vi "Polynomial_Fit.vi"(6 "tolerance":dbl=0.0001, 7 "polynomial order":i32=2, 8 "algorithm":T1 items=["SVD", "Givens", "Givens2", "Householder", "LU Decomposition", "Cholesky", "SVD for Rank Deficient H"], 9 "method":T2 items=["Least Square", "Least Absolute Residual", "Bisquare"], 10 "time":dbl[](array[numeric]), 11 "Y":dbl[](array[numeric])) -> (1 "Polynomial Coefficients":dbl[](array[numeric]), 2 "Equation Y(time)":string, 3 "Plot":cluster{"time":dbl[], "P(A)":dbl[]}[](graph))   [LabVIEW 2022 SP3]
uses:
  <vilib>/Analysis/6fits.llb/Curve Fitting Criteria.ctl
  <vilib>/Analysis/6fits.llb/General Linear Fit Algorithm.ctl
  <vilib>/Analysis/polynomials.llb/Polynomial Plot (Samples).vi
  <vilib>/Analysis/NI_AALPro.lvlib
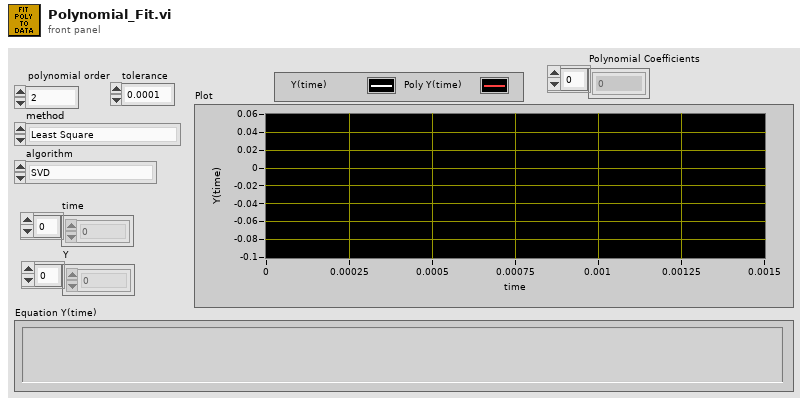
[diagram p1: front panel]
types:
  T1 = typedef "NI_AALPro.lvlib/General Linear Fit Algorithm.ctl" = u16
  T2 = typedef "NI_AALPro.lvlib/Curve Fitting Criteria.ctl" = u16
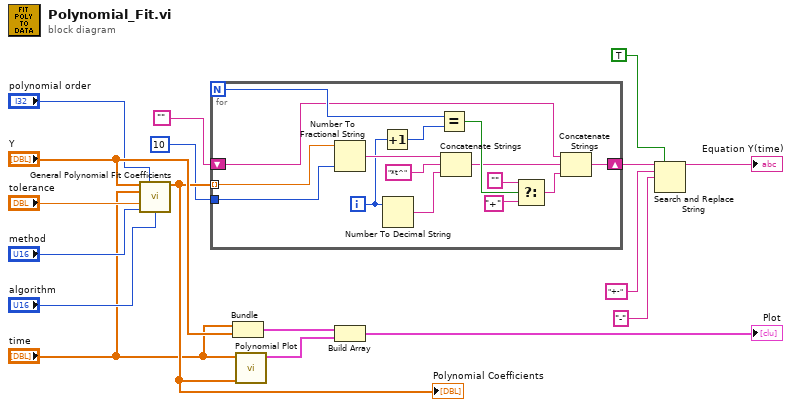
[diagram p0: block diagram]
diagram:
  n1 = call <vilib>:"General Polynomial Fit Coefficients.vi"("Y"="Y", "polynomial order"="polynomial order", "X"="time", "tolerance"="tolerance", "method"="method", "algorithm"="algorithm") -> ("Polynomial Coefficients"=w10:dbl[])  [unwired: 8 in, 1 out]
  "Polynomial Coefficients" <- w10
  n2 = for {
    N -> [w27]
    tunnel: w10 -> [w32] mode=indexing
    tunnel: i16 10 ("precision (6)") -> [w31]
    shift-right: [w23] -> w8
    shift-left: "" -> [w22]
    i -> [w26]
    n3 = Number To Fractional String(number=w32, precision (6)=w31) -> (F-format string=w30:string)  [unwired: 2 in]
    n4 = Increment(x=w26) -> (x+1=w25:i32)
    n5 = Number To Decimal String(number=w26) -> (decimal integer string=w28:string)  [unwired: 1 in]
    n6 = Equal?(x=w27, y=w25) -> (x = y?=w24:bool)
    n7 = Concatenate Strings(w30, "*t^" ("string"), w28) -> (w21:string)
    n8 = Select(t="" ("string"), s=w24, f="+" ("string")) -> (s? t:f=w18:string)
    n9 = Concatenate Strings(w22, w21, w18) -> (w23:string)
  }
  n10 = Bundle("time"="time", "Y"="Y") -> (w16:cluster{"time":dbl[], "Y":dbl[]})  [unwired: 1 in]
  n11 = call-poly <vilib>:"Polynomial Plot.vi"("P(x)"=w10, "X"="time") -> ("polynomial plot"=w15:cluster{dbl[], "P(A)":dbl[]})  [unwired: 8 in, 1 out]
  n12 = Build Array(w16, w15) -> (→"Plot":cluster{"time":dbl[], "P(A)":dbl[]}[])
  n13 = Search and Replace String(replace all?=TRUE ("replace all? (F)"), input string=w8, search string="+-", replace string="-" ("replace string (\"\")")) -> (result string=→"Equation Y(time)":string)  [unwired: 4 in, 3 out]
